vi "Lab2_3Var.vi"() -> ()   [LabVIEW 2022 SP3]
panel:
  out "Led":bool
  out "time":dbl
  in  "Count":bool
  in  "m":i32
  out "S":dbl
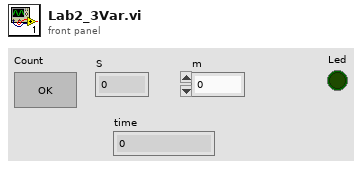
[diagram p1: front panel]
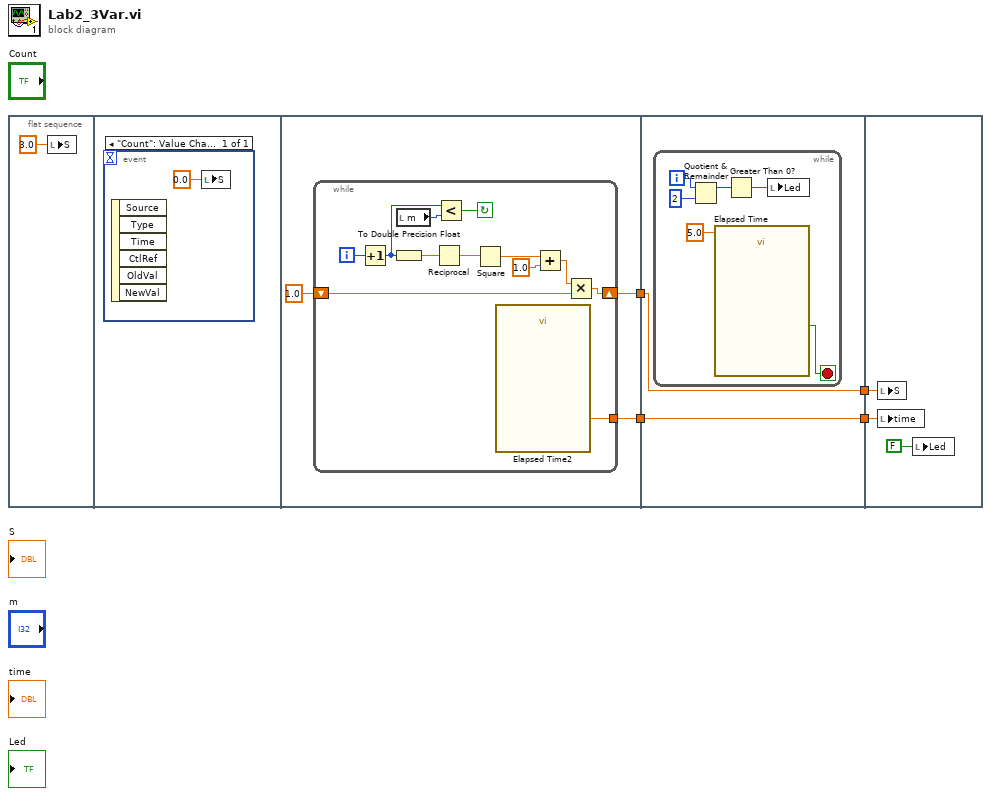
[diagram p0: block diagram]
diagram:
  n1 = flat-sequence {
    tunnel: [w8] -> w3
    tunnel: [w7] -> w1
    tunnel: [w23] -> w4
    tunnel: w3 -> [w23]
    tunnel: [w22] -> w2
    tunnel: w1 -> [w22]
    tunnel: w4 -> [w32]
    tunnel: w2 -> [w30]
    frame #0 {
      n2 = local write "S"(3.0) -> ()
    }
    frame #1 {
      n3 = event shown="[0] \"Count\": Value Change" {
        selector: _ -> [_]
        dyn-events: _ -> [_]
        timeout: _ -> [_]
        event "Count": Value Change {
          n4 = event-data() -> ()  [unwired: 1 in, 6 out]
          n5 = local write "S"(0.0 ("S")) -> ()
        }
      }
    }
    frame #2 {
      n6 = while {
        shift-right: [w11] -> w8
        shift-left: 1.0 -> [w13]
        tunnel: [w10] -> w7
        i -> [w21]
        stop <- w12 continue-if-true
        n7 = Increment(x=w21) -> (x+1=w15:i32)
        n8 = To Double Precision Float(number=w15) -> (double precision float=w20:dbl)
        n9 = local read "m"() -> (w16:i32)
        n10 = Reciprocal(x=w20) -> (1/x=w19:dbl)
        n11 = Less?(x=w15, y=w16) -> (x < y?=w12:bool)
        n12 = Square(x=w19) -> (x^2=w18:dbl)
        n13 = call "Elapsed Time2"() -> ("Elapsed Time (s)"=w10:dbl)  [unwired: 12 in, 7 out]
        n14 = Add(x=w18, y=1.0 ("x+y")) -> (x+y=w14:dbl)
        n15 = Multiply(x=w14, y=w13) -> (x*y=w11:dbl)
      }
    }
    frame #3 {
      n16 = while {
        i -> [w29]
        stop <- w24 stop-if-true
        n17 = Quotient & Remainder(x=w29, y=2 ("floor(x/y)")) -> (x-y*floor(x/y)=w27:i32)  [unwired: 1 out]
        n18 = call "Elapsed Time"("Time Target (s)"=5.0) -> ("Time has Elapsed"=w24:bool)  [unwired: 11 in, 7 out]
        n19 = Greater Than 0?(x=w27) -> (x > 0?=w26:bool)
        n20 = local write "Led"(w26) -> ()
      }
    }
    frame #4 {
      n21 = local write "S"(w32) -> ()
      n22 = local write "time"(w30) -> ()
      n23 = local write "Led"(FALSE) -> ()
    }
  }
